vi "INIT_PCA.vi"(8 "Error In":errorcluster, 11 "LINX Resource 2":T1) -> (0 "error out":errorcluster, 3 "LINX Resource":T1)   [LabVIEW 2026]
uses:
  <vilib>/MakerHub/LINX/Private/Type Defs/LINX Ref.ctl
  <vilib>/MakerHub/LINX/Private/Type Defs/Platform.ctl
  <vilib>/MakerHub/LINX/Private/Type Defs/Interface.ctl
  <vilib>/MakerHub/LINX/Private/Device/Type Defs/LINX Device Config.ctl
  <vilib>/MakerHub/LINX/Private/Device/Type Defs/TCP Config.ctl
  <vilib>/MakerHub/LINX/Private/Device/Type Defs/Channels.ctl
  <vilib>/MakerHub/LINX/Private/Local IO/LinxI2cWrite.vi
  <vilib>/MakerHub/LINX/Public/Utilities/Check Channel.vi
  <vilib>/MakerHub/LINX/Private/Utilties/Generate Error.vi
  <vilib>/MakerHub/LINX/LMH-LINX.lvlib
  <vilib>/MakerHub/LINX/Private/Device/Device.lvlib
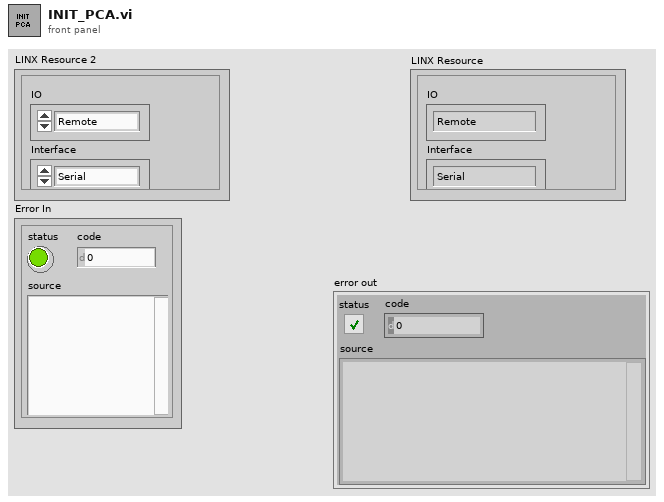
[diagram p1: front panel]
types:
  T1 = typedef "LMH-LINX.lvlib/LINX Ref.ctl" = cluster{"IO":T2, "Interface":T3, "LINX Device Config":T4}
  T2 = typedef "LMH-LINX.lvlib/Platform.ctl" = enum16{"Remote", "Local"}
  T3 = typedef "LMH-LINX.lvlib/Interface.ctl" = enum16{"Serial", "TCP"}
  T4 = typedef "LMH-LINX.lvlib/Device.lvlib/LINX Device Config.ctl" = cluster{"Interface":T3, "COM Port":refnum<visa-resource-name>, "TCP Configuration":T5, "Device Family":u8, "Device ID":u8, "Device Name":string, "TCP Ref":refnum<k5>, "Channels":T6}
  T5 = typedef "LMH-LINX.lvlib/Device.lvlib/TCP Config.ctl" = cluster{"IP Address":string, "Port":u16}
  T6 = typedef "LMH-LINX.lvlib/Channels.ctl" = cluster{"DI":u8[], "DO":u8[], "AI":u8[], "AO":u8[], "PWM":u8[], "QE":u8[], "UART":u8[], "I2C 2":u8[], "SPI":u8[], "CAN":u8[], "Servo":u8[], "AI Ref (V)":dbl, "AI Resolution (Bits)":u8, "AO Ref (V)":dbl, "AO Resolution (Bits)":u8}
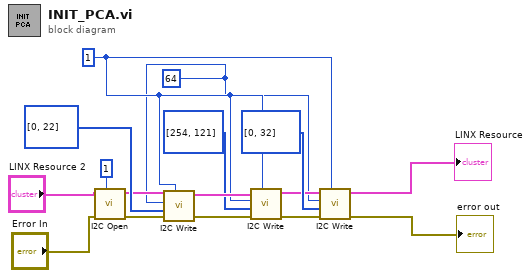
[diagram p0: block diagram]
diagram:
  w4 = u8 64
  w5 = u8 1 ("I2C Channel (0)")
  n1 = call <vilib>:"I2C Open.vi"("I2C Channel (0)"=u8 1, "Error In"="Error In", "LINX Resource"="LINX Resource 2") -> ("Error Out"=w13:errorcluster, "LINX Resource"=w12:T1)  [unwired: 7 in]
  n2 = call <vilib>:"I2C Write.vi"("I2C Channel"=w5, "Error In"=w13, "Data"=u8[] [0, 22], "I2C Slave Address (0)"=w4, "LINX Resource"=w12) -> ("Error Out"=w15:errorcluster, "LINX Resource"=w14:T1)  [unwired: 5 in]
  n3 = call <vilib>:"I2C Write.vi"("I2C Channel"=w5, "Error In"=w15, "Data"=u8[] [254, 121], "I2C Slave Address (0)"=w4, "LINX Resource"=w14) -> ("Error Out"=w11:errorcluster, "LINX Resource"=w6:T1)  [unwired: 5 in]
  n4 = call <vilib>:"I2C Write.vi"("I2C Channel"=w5, "Error In"=w11, "Data"=u8[] [0, 32], "I2C Slave Address (0)"=w4, "LINX Resource"=w6) -> ("Error Out"=→"error out":errorcluster, "LINX Resource"=→"LINX Resource":T1)  [unwired: 5 in]
